vi "FlatToRichrfcontrol_SetMaxTriggerLengthRequest.vi"(5 "OutputClusterType":T1, 11 "InputCluster":T2) -> (3 "OutputCluster":T1)   [LabVIEW 2024, in "FlexSDR_gRPC_client.lvlib"]
uses:
  rfcontrol_SetMaxTriggerLengthRequest_Flat.ctl
  rfcontrol_SetMaxTriggerLengthRequest.ctl
  FlexSDR_gRPC_client.lvlib
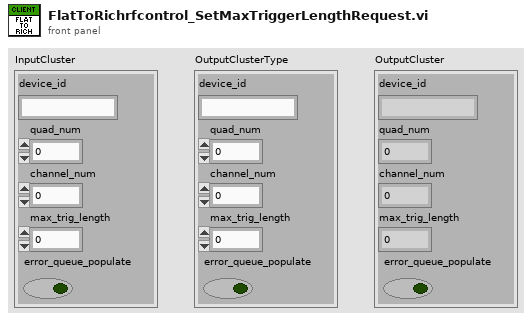
[diagram p1: front panel]
types:
  T1 = typedef "FlexSDR_gRPC_client.lvlib/rfcontrol_SetMaxTriggerLengthRequest.ctl" = cluster{"device_id":string, "quad_num":i32, "channel_num":i32, "max_trig_length":i32, "error_queue_populate":bool}
  T2 = typedef "FlexSDR_gRPC_client.lvlib/rfcontrol_SetMaxTriggerLengthRequest_Flat.ctl" = cluster{"device_id":string, "quad_num":i32, "channel_num":i32, "max_trig_length":i32, "error_queue_populate":bool}
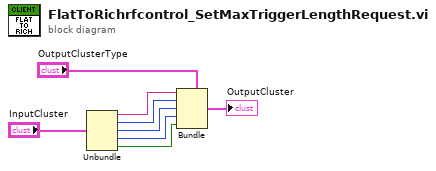
[diagram p0: block diagram]
diagram:
  n1 = Unbundle "Unbundle"("InputCluster") -> ("device_id"=w5:string, "quad_num"=w4:i32, "channel_num"=w3:i32, "max_trig_length"=w2:i32, "error_queue_populate"=w1:bool)
  n2 = Bundle "Bundle"(cluster="OutputClusterType", "device_id"=w5, "quad_num"=w4, "channel_num"=w3, "max_trig_length"=w2, "error_queue_populate"=w1) -> (→"OutputCluster":T1)
